vi "IMUComplementaryFilter.vi"(1 "tau acc":dbl=0.4, 2 "tau mag":dbl=0.05, 5 "Gyro":T3, 7 "Accel":T2, 9 "Mag":T1, 12 "Tilt Comp (Yaw)":bool) -> (4 "Roll":dbl(knob) scale=-180.0..180.0, 6 "Pitch":dbl(knob) scale=-90.0..90.0, 8 "Yaw":dbl(knob) scale=-180.0..180.0)   [LabVIEW 2014]
doc: "Resets the gyroscope to a heading of zero. Use this VI to recalibrate the gyroscope after significant drift.\n\nThis software is licensed. Open the labview\\readme\\WPI Robotics Library Open Source License.txt file for more information."
uses:
  Gyro.ctl
  Accel.ctl
  Mag.ctl
panel:
  # "Yaw tilt compensation should be off when used\nin control loops, as testing reveals that the\naccelerometers negatively affect the dynamic\nperformance of this Yaw output (generates\novershoot in the response).  This is caused by\nthe accelerometers sensing movement in\naddition to gravity, which causes error in the tilt\ncompensation algorithm.  In this case, Yaw will\nonly be accurate when robot/sensor is level.\n\nEnabling Yaw tilt compensation improves yaw\naccuracy when robot is tilted (Pitch or Roll), but\nis only useful when system is static (not moving).\n\nBoth settings should result in drift-free rotation\nindications (Roll/Pitch/Yaw) with the proper\nselection of tau-acc and tau-mag."
  # "When Sensor oriented with positive X-axis\npointing forward, and positive Y-axis\npointing left, and positive Z axis pointing up :\n\nRoll is rotation about X-axis, clockwise roll,\n(looking in + X direction), is positive.\n\nPitch is rotation about Y-axis, clockwise pitch\n(looking in + Y direction), is positive.\n\nYaw is rotation about Z-axis, clockwise yaw\n(looking in + Z direction), is positive."
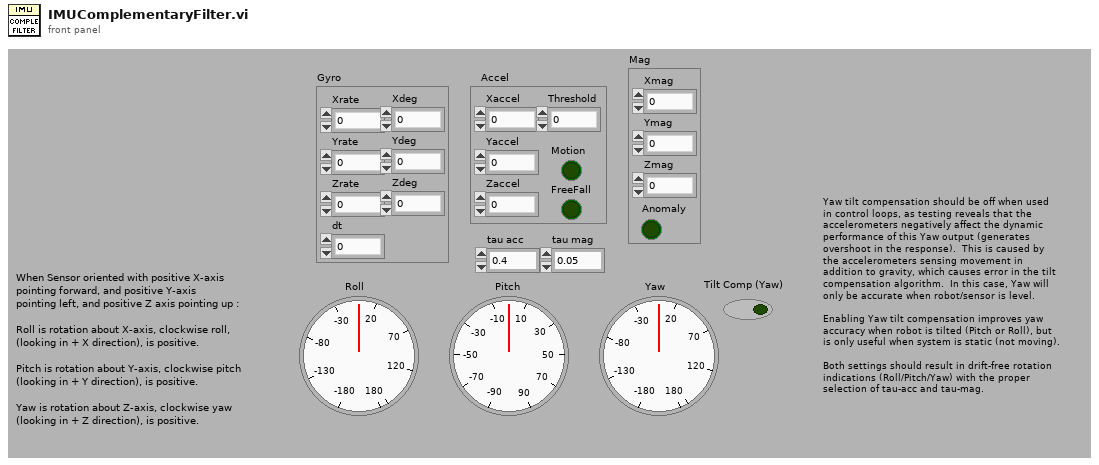
[diagram p1: front panel]
types:
  T1 = typedef "Mag.ctl" = cluster{"Xmag":dbl, "Ymag":dbl, "Zmag":dbl, "Anomaly":bool}
  T2 = typedef "Accel.ctl" = cluster{"Xaccel":dbl, "Yaccel":dbl, "Zaccel":dbl, "Motion":bool, "Threshold":dbl, "FreeFall":bool}
  T3 = typedef "Gyro.ctl" = cluster{"Xrate":dbl, "Yrate":dbl, "Zrate":dbl, "Xdeg":dbl, "Ydeg":dbl, "Zdeg":dbl, "dt":dbl}
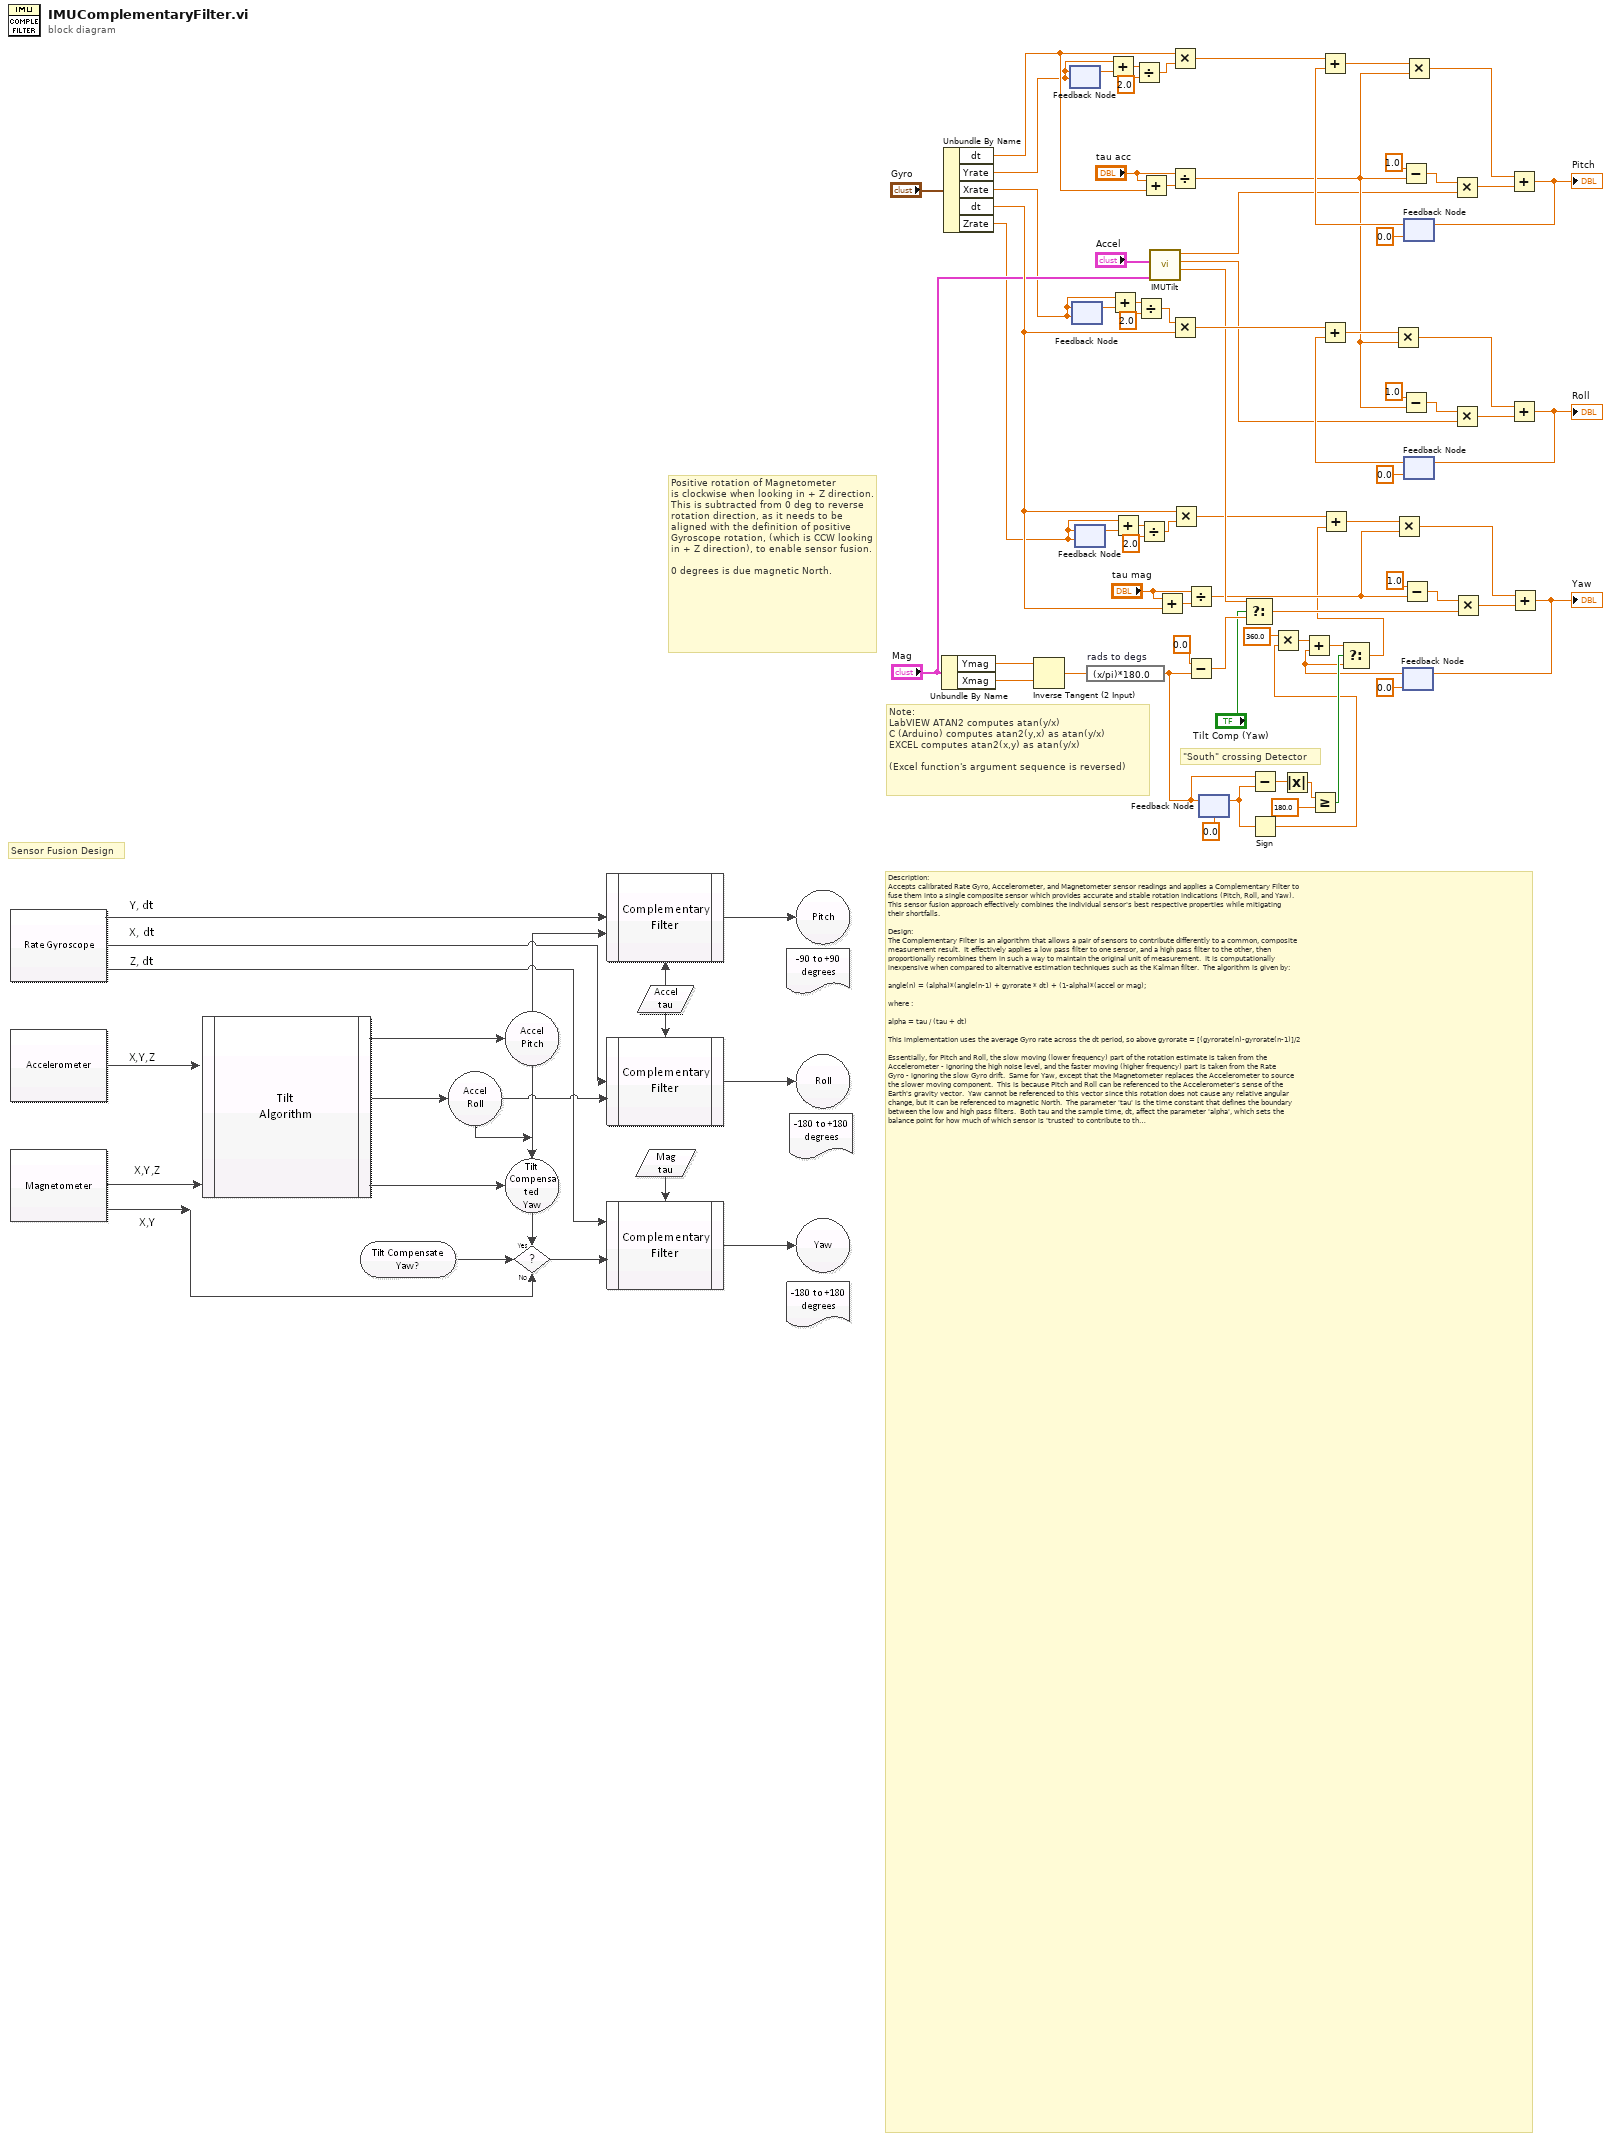
[diagram p0: block diagram]
diagram:
  # "Sensor Fusion Design"
  # "Description:\nAccepts calibrated Rate Gyro, Accelerometer, and Magnetometer sensor readings and applies a Complementary Filter to\nfuse them into a single composite sensor which provides accurate and stable rotation indications (Pitch, Roll, and Yaw).\nThis sensor fusion approach effectively combines the individual sensor's best respective properties while mitigating\ntheir shortfalls.\n\nDesign:\nThe Complementary Filter is an algorithm that allows a pair of sensors to contribute differently to a common, composite\nmeasurement result.  It effectively applies a low pass filter to one sensor, and a high pass filter to the other, then\nproportionally recombines them in such a way to maintain the original unit of measurement.  It is computationally\ninexpensive when compared to alternative estimation techniques such as the Kalman filter.  The algorithm is given by:\n\nangle(n) = (alpha)*(angle(n-1) + gyrorate * dt) + (1-alpha)*(accel or mag);\n\nwhere : \n\nalpha = tau / (tau + dt)\n\nThis implementation uses the average Gyro rate across the dt period, so above gyrorate = [(gyrorate(n)-gyrorate(n-1)]/2\n\nEssentially, for Pitch and Roll, the slow moving (lower frequency) part of the rotation estimate is taken from the\nAccelerometer - ignoring the high noise level, and the faster moving (higher frequency) part is taken from the Rate \nGyro - ignoring the slow Gyro drift.  Same for Yaw, except that the Magnetometer replaces the Accelerometer to source\nthe slower moving component.  This is because Pitch and Roll can be referenced to the Accelerometer's sense of the\nEarth's gravity vector.  Yaw cannot be referenced to this vector since this rotation does not cause any relative angular\nchange, but it can be referenced to magnetic North.  The parameter 'tau' is the time constant that defines the boundary\nbetween the low and high pass filters.  Both tau and the sample time, dt, affect the parameter 'alpha', which sets the\nbalance point for how much of which sensor is 'trusted' to contribute to the rotation estimate.\n\nThe Complementary Filter algorithm is applied to each X/Y/Z rotation axis to compute R/P/Y outputs, respectively.\n\nMagnetometer readings are tilt-compensated when Tilt-Comp-(Yaw) is asserted (True), by the IMU TILT subVI.  This\ncreates what is known as a tilt-compensated compass, which allows Yaw to be insensitive to the effects of a\nnon-level sensor, but generates error in Yaw during movement (coordinate acceleration).\n\nThe Yaw \"South\" crossing detector is necessary to allow a smooth transition across the +/- 180 deg discontinuity (inherent\nin the ATAN function).  Since -180 deg is congruent with +180 deg, Yaw needs to jump between these values when\ncrossing South (North is 0 deg).  The design depends upon comparison of successive Yaw readings to detect a cross-over\nevent.  The cross-over detector monitors the current reading and evaluates how far it is from the previous reading.  If it\nis greater than the previous reading by the Discriminant (= 180 deg), then Yaw just crossed South.\n\nBy choosing 180 as the Discriminant, the only way the detector can produce a false positive, assuming a loop iteration\nof 70 msec, is for it to rotate >2,571 dps ... (2,571=180/.07).  This is faster than the ST L3GD20 Gyro can register.  The\ndetector produces a Boolean True upon detecting a South crossing.  This is used to alter the (n-1) Yaw which was\npreviously stored, either adding or subtracting 360 degrees as required to place the previous Yaw in the correct quadrant\nwhenever crossing occurs.  The Modulus function cannot be used here as the Complementary Filter algorithm has 'state'\n(needs to remember previous Yaw).\n \nWe are in effect stitching together two ends of a ruler for 'modular arithmetic' (clock math).\n\nInputs:\nGYRO - Gyro rate and sample time measurements.\nACCEL - Acceleration measurements.\nMAG - Magnetic measurements.\nTAU ACC - tau parameter used to set sensor balance between Accel and Gyro for Roll and Pitch.\nTAU MAG -  tau parameter used to set sensor balance between Mag and Gyro for Yaw.\nTILT COMP (Yaw) - Enables Yaw tilt-compensation if True.\n\nOutputs:\nROLL - Filtered Roll about sensor X-axis.\nPITCH - Filtered Pitch about sensor Y-axis.\nYAW - Filtered Yaw about sensor Z-axis.\n\nVI Properties:\nExecution Reentrancy is set to Non Reentrant Execution\n\nImplementation:\nIt's best to establish the optimum loop sample time first.  See IMU READ implementation notes for guidance.  Each\ntau parameter should then be adjusted to achieve optimum sensor fusion.  tau acc affects Roll and Pitch, tau mag affects\nYaw.  Start at value 1 or 2 and decrease by half each time until the result doesn't drift, but not so far that the result gets\nnoisy.  An optimum tau for this IMU is likely in the range of 1.0 to 0.01, for a loop sample time between 10 and 100 ms.\n\nNote that both sample timing (dt) and tau both affect the balance parameter, 'alpha'.  Adjusting either dt or tau will\nrequire the other to be readjusted to maintain a particular filter performance.\n\nIt is likely best to set Yaw tilt-compensation to off (False) if the Yaw value is to be used as feedback in a closed loop\ncontrol application.  The tradeoff is that Yaw will only be accurate while the robot is level.\n\nSince a Yaw of -180 degrees is congruent with +180 degrees (they represent the same direction), it is possible that the\nYaw output will oscillate between these two values when the sensor happens to be pointing due South, as sensor\nnoise causes slight variation.  You will need to account for this possibility if you are using the Yaw value for decision-\nmaking in code.\n\n----- The RoboBees FRC Team 836! -----  Complement your passion to solve problems with a STEM Education!"
  # "\"South\" crossing Detector"
  # "Positive rotation of Magnetometer\nis clockwise when looking in + Z direction.  This is subtracted from 0 deg to reverse rotation direction, as it needs to be aligned with the definition of positive Gyroscope rotation, (which is CCW looking in + Z direction), to enable sensor fusion.\n\n0 degrees is due magnetic North."
  # "Note:\nLabVIEW ATAN2 computes atan(y/x)\nC (Arduino) computes atan2(y,x) as atan(y/x)\nEXCEL computes atan2(x,y) as atan(y/x)\n\n(Excel function's argument sequence is reversed)"
  n1 = Unbundle By Name("Mag") -> ("Ymag"=w42:dbl, "Xmag"=w41:dbl)
  n2 = Unbundle By Name("Gyro") -> ("dt"=w52:dbl, "Yrate"=w24:dbl, "Xrate"=w18:dbl, "dt"=w43:dbl, "Zrate"=w13:dbl)
  n3 = Inverse Tangent (2 Input)(1:w41, 2:w42) -> (0:w40:dbl)
  n4 = feedback #1(w24) -> (w26:dbl)
  n5 = feedback-in #1(w24) -> ()
  n6 = feedback #2(w18) -> (w19:dbl)
  n7 = feedback-in #2(w18) -> ()
  n8 = feedback #3(w13) -> (w16:dbl)
  n9 = feedback-in #3(w13) -> ()
  n10 = expression code="(x/pi)*180.0" "rads to degs"(w40) -> (w3:dbl)
  n11 = Add(x=w24, y=w26) -> (x+y=w25:dbl)
  n12 = Add(x=w18, y=w19) -> (x+y=w20:dbl)
  n13 = Add(x=w13, y=w16) -> (x+y=w15:dbl)
  n14 = Divide(x=w25, y=2.0) -> (x/y=w22:dbl)
  n15 = Divide(x=w20, y=2.0) -> (x/y=w17:dbl)
  n16 = Divide(x=w15, y=2.0) -> (x/y=w12:dbl)
  n17 = Add(x="tau acc", y=w52) -> (x+y=w74:dbl)
  n18 = call "IMUTilt.vi"("Mag"="Mag", "Accel"="Accel") -> ("Yaw"=w33:dbl, "Roll"=w34:dbl, "Pitch"=w54:dbl)  [unwired: 6 in]
  n19 = Add(x="tau mag", y=w43) -> (x+y=w44:dbl)
  n20 = Multiply(x=w52, y=w22) -> (x*y=w62:dbl)
  n21 = Divide(x="tau acc", y=w74) -> (x/y=w58:dbl)
  n22 = Multiply(x=w17, y=w43) -> (x*y=w72:dbl)
  n23 = Multiply(x=w43, y=w12) -> (x*y=w31:dbl)
  n24 = Divide(x="tau mag", y=w44) -> (x/y=w30:dbl)
  n25 = Subtract(x=0.0 ("y"), y=w3) -> (x-y=w36:dbl)
  n26 = feedback-in #4(w3) -> ()
  n27 = feedback #4(0.0) -> (w4:dbl)
  n28 = Select(t=w33, s="Tilt Comp (Yaw)", f=w36) -> (s? t:f=w37:dbl)
  n29 = Subtract(x=w3, y=w4) -> (x-y=w10:dbl)
  n30 = Sign(1:w4) -> (0:w6:dbl)
  n31 = Multiply(x=360.0 ("y"), y=w6) -> (x*y=w2:dbl)
  n32 = Absolute Value(x=w10) -> (abs(x)=w9:dbl)
  n33 = Greater Or Equal?(x=w9, y=180.0) -> (x >= y?=w7:bool)
  n34 = Subtract(x=1.0, y=w58) -> (x-y=w61:dbl)
  n35 = Subtract(x=1.0, y=w58) -> (x-y=w57:dbl)
  n36 = Subtract(x=1.0, y=w30) -> (x-y=w50:dbl)
  n37 = feedback #5(0.0) -> (w1:dbl)
  n38 = Add(x=w2, y=w1) -> (x+y=w27:dbl)
  n39 = Select(t=w27, s=w7, f=w1) -> (s? t:f=w28:dbl)
  n40 = Add(x=w31, y=w28) -> (x+y=w47:dbl)
  n41 = Multiply(x=w47, y=w30) -> (x*y=w49:dbl)
  n42 = feedback #6(0.0) -> (w66:dbl)
  n43 = Add(x=w62, y=w66) -> (x+y=w63:dbl)
  n44 = Multiply(x=w63, y=w58) -> (x*y=w65:dbl)
  n45 = feedback #7(0.0) -> (w53:dbl)
  n46 = Add(x=w72, y=w53) -> (x+y=w71:dbl)
  n47 = Multiply(x=w71, y=w58) -> (x*y=w69:dbl)
  n48 = Multiply(x=w61, y=w54) -> (x*y=w64:dbl)
  n49 = Multiply(x=w57, y=w34) -> (x*y=w70:dbl)
  n50 = Multiply(x=w50, y=w37) -> (x*y=w48:dbl)
  n51 = Add(x=w65, y=w64) -> (x+y=w55:dbl)
  "Pitch" <- w55
  n52 = feedback-in #6(w55) -> ()
  n53 = Add(x=w69, y=w70) -> (x+y=w56:dbl)
  "Roll" <- w56
  n54 = feedback-in #7(w56) -> ()
  n55 = Add(x=w49, y=w48) -> (x+y=w11:dbl)
  "Yaw" <- w11
  n56 = feedback-in #5(w11) -> ()
